vi "Define 2D Helmholtz PDE Domain (Rect).vi"(0 "PDE in":refnum<class "NI_PDE.lvclass">, 5 "X":T2={"start x"=0.0, "end x"=1.0, "# of x-points"=11}, 7 "Y":T1={"start y"=0.0, "end y"=1.0, "# of y-points"=11}, 11 "error in (no error)":errorcluster) -> (4 "PDE out":refnum<class "NI_PDE.lvclass">, 15 "error out":errorcluster)   [LabVIEW 2020, in "NI_PDE.lvlib"]
doc: "Defines the domain where you solve the partial differential equation. You must manually select the polymorphic instance to use."
uses:
  <vilib>/gmath/NI_PDE.lvlib
  <vilib>/gmath/pde.llb/PDEClass/NI_PDE.lvclass
  <vilib>/gmath/pde.llb/PDEClass/PDE_Helmholtz_2D/NI_PDE_Helmholtz_2D.lvclass
  e:/builds/penguin/labview/branches/2020/dev/dist/vi.lib/gmath/pde.llb/PDEClass/NI_PDE.lvclass
  <vilib>/gmath/pde.llb/DomainClass/Domain_Steady_2D_Rect/NI_Domain_Steady_2D_Rect.lvclass
  e:/builds/penguin/labview/branches/2020/dev/dist/vi.lib/gmath/pde.llb/DomainClass/NI_Domain.lvclass
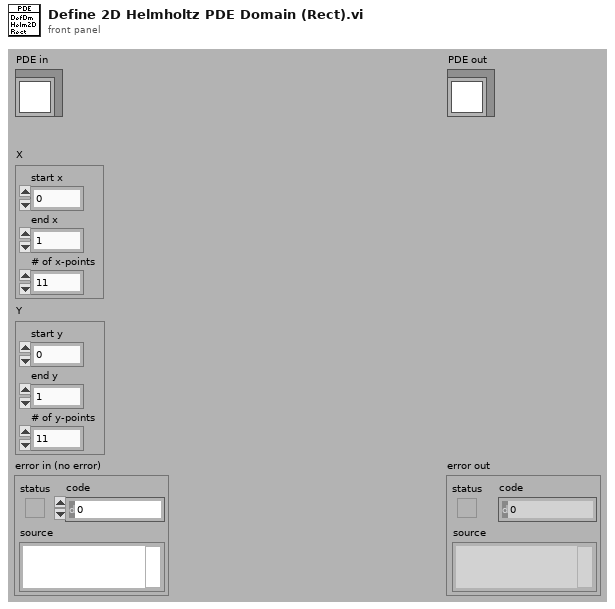
[diagram p1: front panel]
types:
  T1 = cluster{"start y":dbl, "end y":dbl, "# of y-points":i32}
  T2 = cluster{"start x":dbl, "end x":dbl, "# of x-points":i32}
  T3 = cluster{"X":cluster{"start x":dbl, "end x":dbl, "# of x-points":i32}, "Y":cluster{"start y":dbl, "end y":dbl, "# of y-points":i32}}
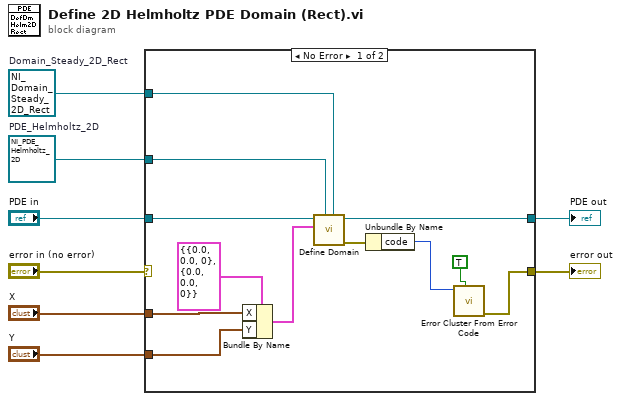
[diagram p0: block diagram]
diagram:
  w1 = refnum<class "NI_Domain_Steady_2D_Rect.lvclass"> refnum  # Domain_Steady_2D_Rect
  w2 = refnum<class "NI_PDE_Helmholtz_2D.lvclass"> refnum  # PDE_Helmholtz_2D
  n1 = case shown="No Error" "error in (no error)" {
    selector: "error in (no error)" -> [_ w22]
    tunnel: "PDE in" -> [w14 w21]
    tunnel: [w11 w21] -> w7
    tunnel: "Y" -> [w15 _]
    tunnel: "X" -> [w16 _]
    tunnel: [w18 w22] -> w4
    tunnel: w2 -> [w13 _]
    tunnel: w1 -> [w12 _]
    frame No Error {
      n2 = Bundle By Name(cluster=T3 {"X"={"start x"=0.0, "end x"=0.0, "# of x-points"=0}, "Y"={"start y"=0.0, "end y"=0.0, "# of y-points"=0}} ("domain data"), "X"=w16, "Y"=w15) -> (w9:T3)
      n3 = call <vilib>:"Define Domain.vi"("target Domain"=w12, "target PDE"=w13, "domain"=w9, "PDE in"=w14) -> ("error out"=w10:errorcluster, "PDE out"=w11:refnum<class "NI_PDE.lvclass">)  [unwired: 1 in, 5 out]
      n4 = Unbundle By Name(w10) -> ("code"=w20:i32)
      n5 = call <vilib>:"Error Cluster From Error Code.vi"("show call chain? (False)"=TRUE, "error code (0)"=w20) -> ("error out"=w18:errorcluster)  [unwired: 1 in, 6 out]
    }
    frame Error {
    }
  }
  "PDE out" <- w7
  "error out" <- w4
